vi "PortCommunicationSubVI.vi"(4 "Value":string, 5 "VISA Refnum in":refnum<visa-resource-name>) -> (0 "error out":errorcluster, 2 "read buffer":string)   [LabVIEW 2012]
uses:
  <vilib>/Instr/_visa.llb/VISA Configure Serial Port (Instr).vi
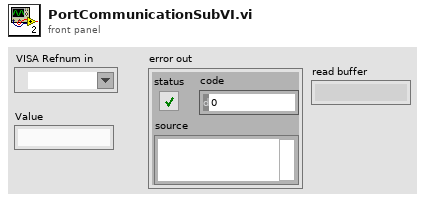
[diagram p1: front panel]
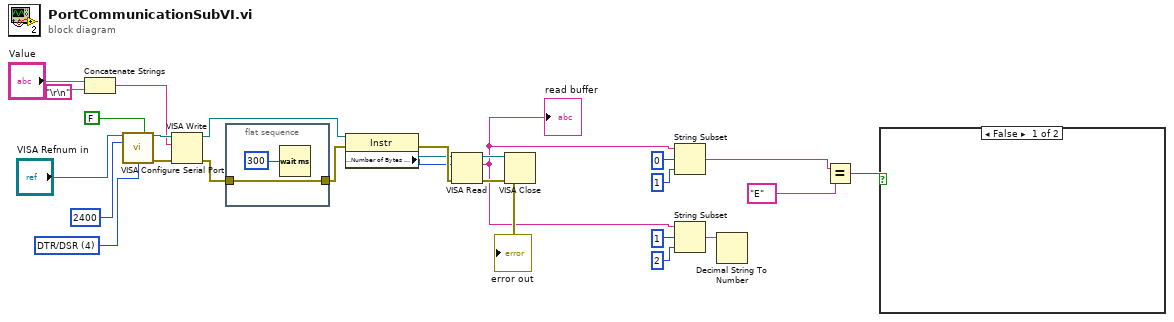
[diagram p0: block diagram]
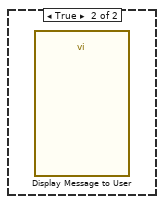
[diagram p2: hidden frame]
diagram:
  w25 = u16 4 items=["None", "XON/XOFF", "RTS/CTS", "XON/XOFF & RTS/CTS", "DTR/DSR", "XON/XOFF & DTR/DSR"] ("flow control (0:none)")
  n1 = Concatenate Strings("Value", "\r\n") -> (w19:string)
  n2 = call-poly "VISA Configure Serial Port"("VISA resource name"="VISA Refnum in", "Enable Termination\nChar (T)"=FALSE ("Enable Termination\nChar (T)"), "baud rate (9600)"=u32 2400, "flow control (0:none)"=w25) -> ("VISA resource name out"=w23:refnum<visa-resource-name>, "error out"=w22:errorcluster)  [unwired: 10 in]
  n3 = VISA Write(VISA resource name=w23, write buffer=w19, error in (no error)=w22) -> (VISA resource name out=w12:refnum<visa-resource-name>, error out=w11:errorcluster)  [unwired: 1 out]
  n4 = flat-sequence {
    tunnel: w11 -> [w29]
    tunnel: [w29] -> w17
    frame #0 {
      n5 = Wait (ms)(milliseconds to wait=u32 300) -> ()  [unwired: 1 out]
    }
  }
  n6 = property class="Instr"(reference=w12, error in=w17) -> (reference out=w13:refnum<visa-resource-name>, error out=w15:errorcluster, "Serial Settings:Number of Bytes at Serial Port"=w14:u32)
  n7 = VISA Read(VISA resource name=w13, byte count=w14, error in (no error)=w15) -> (VISA resource name out=w16:refnum<visa-resource-name>, read buffer=w1:string, error out=w18:errorcluster)  [unwired: 1 out]
  "read buffer" <- w1
  n8 = VISA Close(VISA resource name=w16, error in (no error)=w18) -> (error out=→"error out":errorcluster)
  n9 = String Subset(string=w1, offset (0)=0, length (rest)=1 ("length (rest)")) -> (substring=w4:string)
  n10 = String Subset(string=w1, offset (0)=1, length (rest)=2 ("length (rest)")) -> (substring=w7:string)
  n11 = Decimal String To Number(string=w7) -> ()  [unwired: 2 in, 2 out]
  n12 = Equal?(x=w4, y="E") -> (x = y?=w2:bool)
  n13 = case shown="False" w2 {
    frame False {
    }
    frame True {
      n14 = call "Display Message to User"() -> ()  [unwired: 10 in, 2 out]
    }
  }
